vi "write_sub_pend_fw3.vi"(7 "instance":i32, 8 "pendMotorVal":u16 max=1023, 9 "pendDir":bool=TRUE, 11 "enableWrite":bool=TRUE) -> ()   [LabVIEW 2023]
uses:
  LVLib/SADI_FW3.lvlib
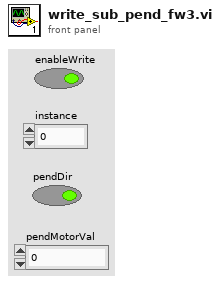
[diagram p1: front panel]
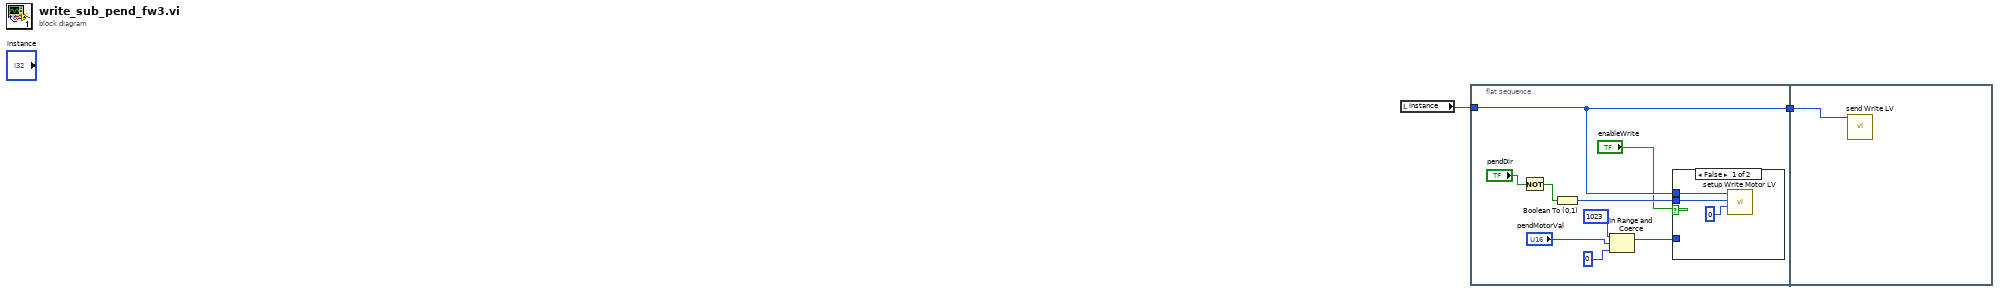
[diagram p0: block diagram]
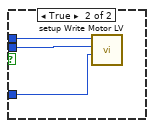
[diagram p2: hidden frame]
diagram:
  n1 = local read "instance"() -> (w1:i32)
  n2 = flat-sequence {
    tunnel: [w11] -> w2
    tunnel: w1 -> [w11]
    tunnel: w2 -> [w18]
    frame #0 {
      n3 = Not(x="pendDir") -> (.not. x?=w3:bool)
      n4 = Boolean To (0,1)(Boolean=w3) -> (0, 1=w10:i16)
      n5 = In Range and Coerce(upper limit=u16 1023, x="pendMotorVal", lower limit=u16 0) -> (coerced(x)=w9:u16)  [unwired: 1 out]
      n6 = case shown="False" "enableWrite" {
        tunnel: w11 -> [w14 w17]
        tunnel: w10 -> [w13 w16]
        tunnel: w9 -> [_ w15]
        frame False {
          n7 = call "setup Write Motor LV.vi"("value"=u16 0, "motorNum"=w13, "instance"=w14) -> ()  [unwired: 9 in]
        }
        frame True {
          n8 = call "setup Write Motor LV.vi"("value"=w15, "motorNum"=w16, "instance"=w17) -> ()  [unwired: 9 in]
        }
      }
    }
    frame #1 {
      n9 = call "send Write LV.vi"("instance"=w18) -> ()  [unwired: 11 in]
    }
  }
